vi "Corr manager.vi"() -> ()   [LabVIEW 2019]
uses:
  Global CORR.vi
  Global percorso impostazioni.vi
  <vilib>/Utility/file.llb/Write Delimited Spreadsheet (DBL).vi
  <vilib>/Utility/file.llb/Read Delimited Spreadsheet (string).vi
panel:
  in  "EXIT":bool
  in  "carica":bool
  in  "Save Button":bool
  in  "coeff correz":T1={"H1 (QH)"=1.0, "H2 (QH)"=1.0, "H1 (NPSH)"=1.0, "H2 (NPSH)"=1.0, "Abilita\\disabilita"=FALSE}
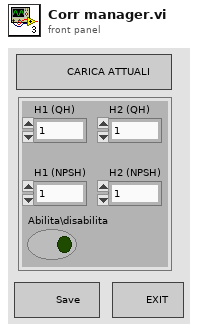
[diagram p1: front panel]
types:
  T1 = cluster{"H1 (QH)":dbl, "H2 (QH)":dbl, "H1 (NPSH)":dbl, "H2 (NPSH)":dbl, "Abilita\\disabilita":bool}
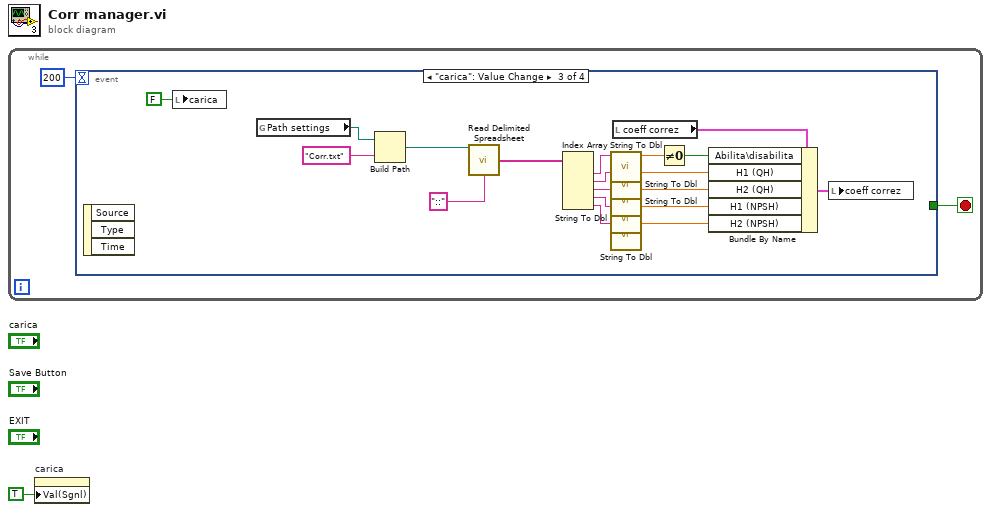
[diagram p0: block diagram]
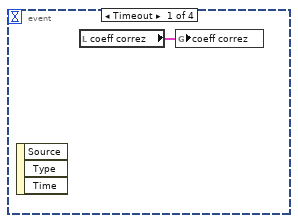
[diagram p2: hidden frame]
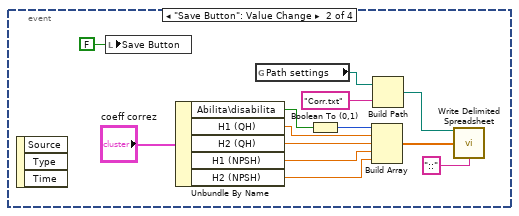
[diagram p3: hidden frame]
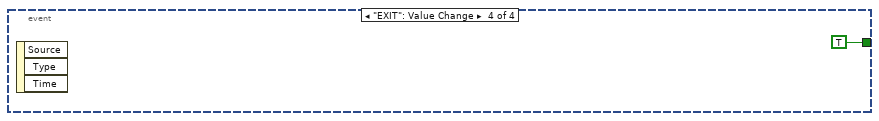
[diagram p4: hidden frame]
diagram:
  n1 = while {
    stop <- w3 stop-if-true
    n2 = event shown="[2] \"carica\": Value Change" {
      selector: _ -> [_ _ _ _]
      dyn-events: _ -> [_ _ _ _]
      timeout: 200 -> [_ _ _ _]
      tunnel: [_ _ _ TRUE] -> w3
      event Timeout {
        n3 = event-data() -> ()  [unwired: 1 in, 3 out]
        n4 = local read "coeff correz"() -> (w4:T1)
        n5 = global write "Global CORR.vi" "coeff correz"(w4) -> ()
      }
      event "Save Button": Value Change {
        n6 = event-data() -> ()  [unwired: 1 in, 3 out]
        n7 = local write "Save Button"(FALSE ("Save Button")) -> ()
        n8 = Unbundle By Name("coeff correz") -> ("Abilita\\disabilita"=w10:bool, "H1 (QH)"=w12:dbl, "H2 (QH)"=w13:dbl, "H1 (NPSH)"=w14:dbl, "H2 (NPSH)"=w15:dbl)
        n9 = global read "Global percorso impostazioni.vi" "Path settings"() -> (w8:path)
        n10 = Boolean To (0,1)(Boolean=w10) -> (0, 1=w11:i16)
        n11 = Build Array(w11, w12, w13, w14, w15) -> (w16:dbl[])
        n12 = Build Path(base path=w8, name or relative path="Corr.txt") -> (appended path=w6:path)
        n13 = call-poly <vilib>:"Write Delimited Spreadsheet.vi"("file path (dialog if empty)"=w6, "1D data"=w16, "delimiter (\\t)"="::" ("delimiter (\\t)")) -> ()  [unwired: 11 in, 2 out]
      }
      event "carica": Value Change {
        n14 = event-data() -> ()  [unwired: 1 in, 3 out]
        n15 = local write "carica"(FALSE ("carica")) -> ()
        n16 = global read "Global percorso impostazioni.vi" "Path settings"() -> (w36:path)
        n17 = Build Path(base path=w36, name or relative path="Corr.txt") -> (appended path=w34:path)
        n18 = call-poly <vilib>:"Read Delimited Spreadsheet.vi"("file path (dialog if empty)"=w34, "delimiter (\\t)"="::" ("delimiter (\\t)")) -> ("first row"=w32:string[])  [unwired: 8 in, 5 out]
        n19 = Index Array(array=w32) -> (element #1=w31:string, element #2=w30:string, element #3=w29:string, element #4=w28:string, element #5=w27:string)  [unwired: 5 in]
        n20 = call "String To Dbl.vi"("String"=w31) -> ("Numeric"=w24:dbl)  [unwired: 10 in]
        n21 = call "String To Dbl.vi"("String"=w30) -> ("Numeric"=w22:dbl)  [unwired: 10 in]
        n22 = call "String To Dbl.vi"("String"=w29) -> ("Numeric"=w21:dbl)  [unwired: 10 in]
        n23 = call "String To Dbl.vi"("String"=w28) -> ("Numeric"=w20:dbl)  [unwired: 10 in]
        n24 = call "String To Dbl.vi"("String"=w27) -> ("Numeric"=w19:dbl)  [unwired: 10 in]
        n25 = local read "coeff correz"() -> (w25:T1)
        n26 = Not Equal To 0?(x=w24) -> (x != 0?=w23:bool)
        n27 = Bundle By Name(cluster=w25, "Abilita\\disabilita"=w23, "H1 (QH)"=w22, "H2 (QH)"=w21, "H1 (NPSH)"=w20, "H2 (NPSH)"=w19) -> (w26:T1)
        n28 = local write "coeff correz"(w26) -> ()
      }
      event "EXIT": Value Change {
        n29 = event-data() -> ()  [unwired: 1 in, 3 out]
      }
    }
  }
  n30 = property on="carica" class="Bool (strict)"("Val(Sgnl)"=TRUE ("Value (Signaling)")) -> ()  [unwired: 2 in, 2 out]
